vi "SetAmbientPressure.vi"(8 "error in (no error)":errorcluster, 9 "Ambient Pressure":sgl, 10 "Address":u8, 11 "VISA resource name":refnum<visa-resource-name>) -> (0 "error out":errorcluster, 1 "Raw Response":string, 3 "VISA resource name out":refnum<visa-resource-name>)   [LabVIEW 2020, in "driver_flodx_pressure.lvlib"]
doc: "Sets the value that of the ambient pressure(used to calculate absolute pressure), please make sure\nthe units(kPa,BAR,PSI) of the value you are sending is matching with the units(kPa,BAR,PSI) the device is using."
uses:
  <instrlib>/RxnRover/FloDx Pressure Driver/driver_flodx_pressure.lvlib
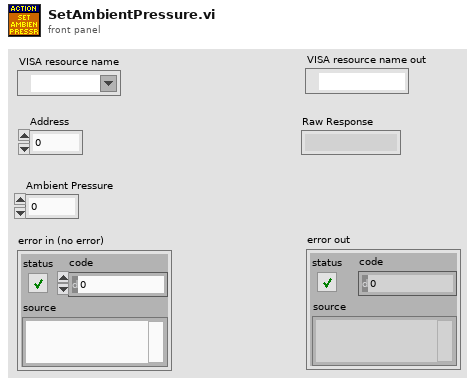
[diagram p1: front panel]
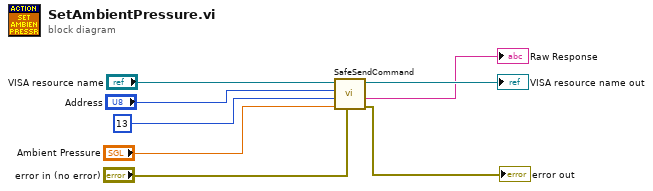
[diagram p0: block diagram]
diagram:
  n1 = call <instrlib>:"SafeSendCommand.vi"("error in"="error in (no error)", "Parameter"="Ambient Pressure", "Command #"=u8 13 ("Command"), "Address #"="Address", "VISA resource name"="VISA resource name") -> ("error out"=→"error out":errorcluster, "Raw Response"=→"Raw Response":string, "VISA resource name out"=→"VISA resource name out":refnum<visa-resource-name>)  [unwired: 3 in, 1 out]
